vi "av.vi"(1 "tango data type":T1=enum."STRING_SPE", 2 "data":u8[](array[numeric])=[0], 3 "dim. y":i32, 4 "dim. x":i32, 5 "attribute name":string, 6 "device name":string) -> (0 "attribute value":T2={"device name"="", "attribute name"="", "quality value"=enum."VALID", "quality string"="", "timestamp"=0.0, "dim. x"=0, "dim. y"=0, "value"=[], "error code"=0, "error stack"=[], "data type"=enum."STRING_SPE"})   [LabVIEW 2014, in "tango.lvlib"]
uses:
  tango.lvlib
  Common VIs/Typedefs/_AttributeValue_t.ctl
  Common VIs/Typedefs/_AttributeQuality_t.ctl
  Common VIs/Typedefs/_AttributeDataType_t.ctl
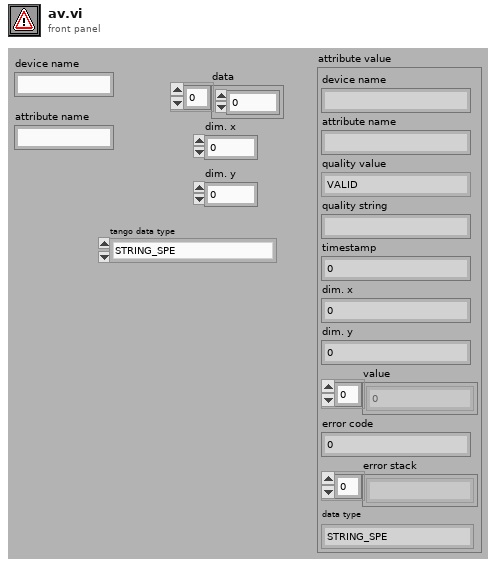
[diagram p1: front panel]
types:
  T1 = typedef "tango.lvlib/_AttributeDataType_t.ctl" = enum16{"STATE_SCA", "STATE_SPE", "STATE_IMG", "STRING_SCA", "STRING_SPE", "STRING_IMG", "BOOL_SCA", "BOOL_SPE", "BOOL_IMG", "UCHAR_SCA", "UCHAR_SPE", "UCHAR_IMG", "SHORT_SCA", "SHORT_SPE", "SHORT_IMG", "USHORT_SCA", "USHORT_SPE", "USHORT_IMG", "LONG_SCA", "LONG_SPE", "LONG_IMG", "ULONG_SCA", "ULONG_SPE", "ULONG_IMG", "LONG64_SCA", "LONG64_SPE", "LONG64_IMG", "ULONG64_SCA", "ULONG64_SPE", "ULONG64_IMG", "FLOAT_SCA", "FLOAT_SPE", "FLOAT_IMG", "DOUBLE_SCA", "DOUBLE_SPE", "DOUBLE_IMG", "UNKNOWN_DATA_TYPE"}
  T2 = typedef "tango.lvlib/_AttributeValue_t.ctl" = cluster{"device name":string, "attribute name":string, "quality value":T3, "quality string":string, "timestamp":dbl, "dim. x":i32, "dim. y":i32, "value":u8[], "error code":i32, "error stack":string[], "data type":T1}
  T3 = typedef "tango.lvlib/_AttributeQuality_t.ctl" = enum16{"VALID", "INVALID", "ALARM", "CHANGING", "UNKNOWN_QUALITY"}
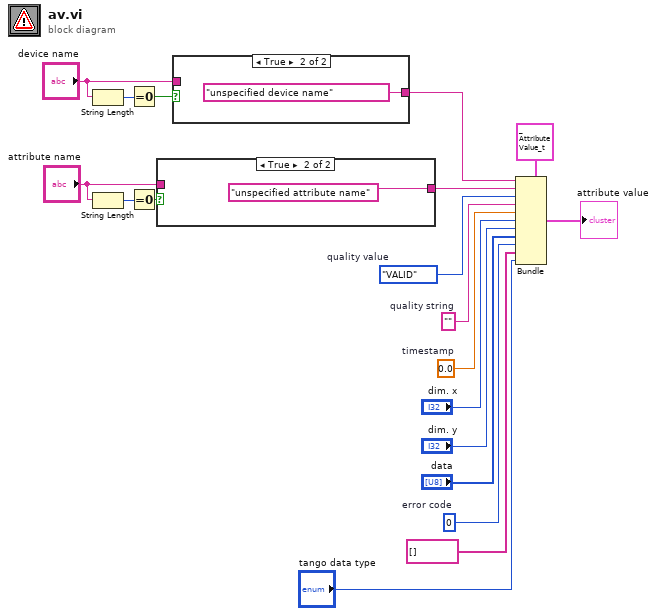
[diagram p0: block diagram]
diagram:
  w19 = 0  # error code
  w15 = 0.0  # timestamp
  w14 = ""  # quality string
  w13 = _AttributeQuality_t."VALID"  # quality value
  n1 = String Length(string="device name") -> (length=w12:i32)
  n2 = String Length(string="attribute name") -> (length=w8:i32)
  n3 = Equal To 0?(x=w12) -> (x = 0?=w11:bool)
  n4 = Equal To 0?(x=w8) -> (x = 0?=w7:bool)
  n5 = case shown="True" w7 {
    tunnel: "attribute name" -> [w20 _]
    tunnel: [w20 "unspecified attribute name" ("attribute name")] -> w5
    frame False {
    }
    frame True {
    }
  }
  n6 = case shown="True" w11 {
    tunnel: "device name" -> [w22 _]
    tunnel: [w22 "unspecified device name" ("device name")] -> w9
    frame False {
    }
    frame True {
    }
  }
  n7 = Bundle(cluster=T2 {"device name"="", "attribute name"="", "quality value"=enum."VALID", "quality string"="", "timestamp"=0.0, "dim. x"=0, "dim. y"=0, "value"=[], "error code"=0, "error stack"=[], "data type"=enum."STRING_SPE"} ("attribute value 2"), "device name"=w9, "attribute name"=w5, "quality value"=w13, "quality string"=w14, "timestamp"=w15, "dim. x"="dim. x", "dim. y"="dim. y", "value"="data", "error code"=w19, "error stack"=string[] [], "data type"="tango data type") -> (→"attribute value":T2)
